vi "can angle lift.vi"(8 "error in (no error)":errorcluster, 10 "Down button":bool, 11 "Up button":bool) -> (0 "error out":errorcluster)   [LabVIEW 2014]
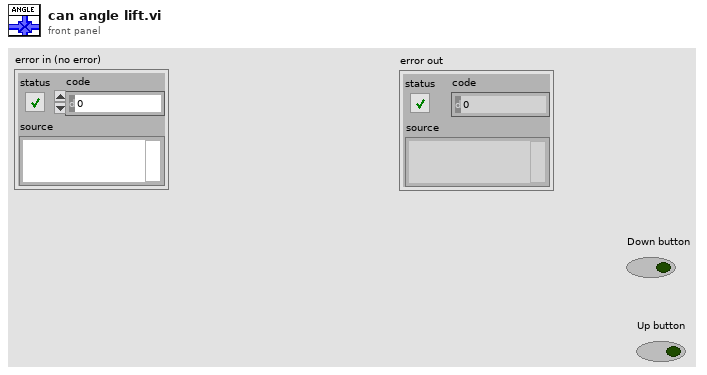
[diagram p1: front panel]
types:
  T1 = typedef "WPI_MotorControlDeviceRef.ctl" = cluster{"DeviceStatus":errorcluster, "Type":T2, "PWM":cluster{"Controller":T3, "PWM Channel":T4, "DeadBand":T5}, "CAN":cluster{"Device Number":u8, "Control Mode":T6, "Semaphore":T7, "Max Vout":dbl, "TalonSRX Control Mode":T8}, "Invert":bool, "TransformRef":T9, "InvTransformRef":T9}
  T2 = typedef "WPI_MotorControlType.ctl" = enum16{"PWM", "CAN", "CANTalonSRX"}
  T3 = typedef "FPGA_TypedefDigitalModule.ctl" = enum16{"Controller 1"}
  T4 = typedef "FPGA_DIOPWMChannel.ctl" = enum8{"PWM 0", "PWM 1", "PWM 2", "PWM 3", "PWM 4", "PWM 5", "PWM 6", "PWM 7", "PWM 8", "PWM 9", "PWM MXP 0", "PWM MXP 1", "PWM MXP 2", "PWM MXP 3", "PWM MXP 4", "PWM MXP 5", "PWM MXP 6", "PWM MXP 7", "PWM MXP 8", "PWM MXP 9", "Invalid"}
  T5 = typedef "WPI_PWMDeadband.ctl" = cluster{"Name":string, "maxPositivePwm":i32, "minPositivePwm":i32, "centerPwm":i32, "maxNegativePwm":i32, "minNegativePwm":i32, "angularRange":u16}
  T6 = typedef "WPI_CANJaguar_ControlMode.ctl" = enum8{"Percent VBus", "Current", "Speed", "Position", "Voltage"}
  T7 = typedef "Semaphore RefNum" = refnum<k1>
  T8 = typedef "WPI_CANTalonSRX_APIControlMode.ctl" = enum8{"Percent VBus", "Speed", "Position", "Slave", "Unchanged / Invalid"}
  T9 = typedef "WPI_PWMTransform_ConPane.ctl" = refnum<vi>
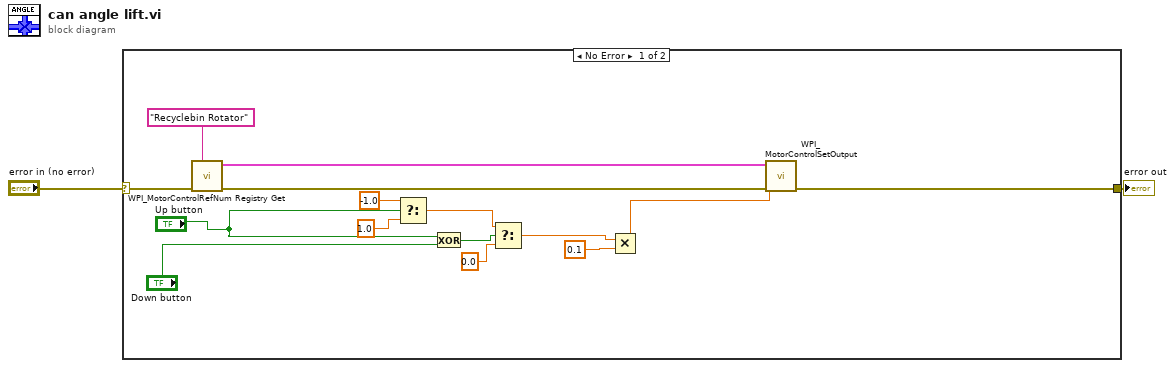
[diagram p0: block diagram]
diagram:
  n1 = case shown="No Error" "error in (no error)" {
    selector: "error in (no error)" -> [w17 w18]
    tunnel: [w3 w18] -> w1
    frame No Error {
      n2 = call <vilib>:"WPI_MotorControlRefNum Registry Get.vi"("error in (no error)"=w17, "refnum name"="Recyclebin Rotator") -> ("error out"=w4:errorcluster, "MotorControlDevRef"=w6:T1)  [unwired: 8 in]
      n3 = Select(t=-1.0, s="Up button", f=1.0) -> (s? t:f=w12:dbl)
      n4 = Exclusive Or(1:"Down button", 2:"Up button") -> (0:w11:bool)
      n5 = Select(t=w12, s=w11, f=0.0) -> (s? t:f=w10:dbl)
      n6 = Multiply(x=w10, y=0.1) -> (x*y=w5:dbl)
      n7 = call <vilib>:"WPI_MotorControlSetOutput.vi"("error in (no error)"=w4, "Output"=w5, "MotorControlDevRef"=w6) -> ("error out"=w3:errorcluster)  [unwired: 6 in, 2 out]
    }
    frame Error {
      # "This is what to do if there is an error.  Usually it is nothing."
    }
  }
  "error out" <- w1
